vi "RUSHArmControl.vi"(1 "In Cluster":T3) -> (0 "Out Cluster":T2)   [LabVIEW 2012]
uses:
  <vilib>/Rock Robotics/WPI/Relay/WPI_RelayValue.ctl
panel:
  in  "Max Speed":dbl=0.5
  in  "Setpoint P Gain":dbl=2.0
  in  "Manual P Gain":dbl=2.0
  in  "Vision P Gain":dbl=0.75
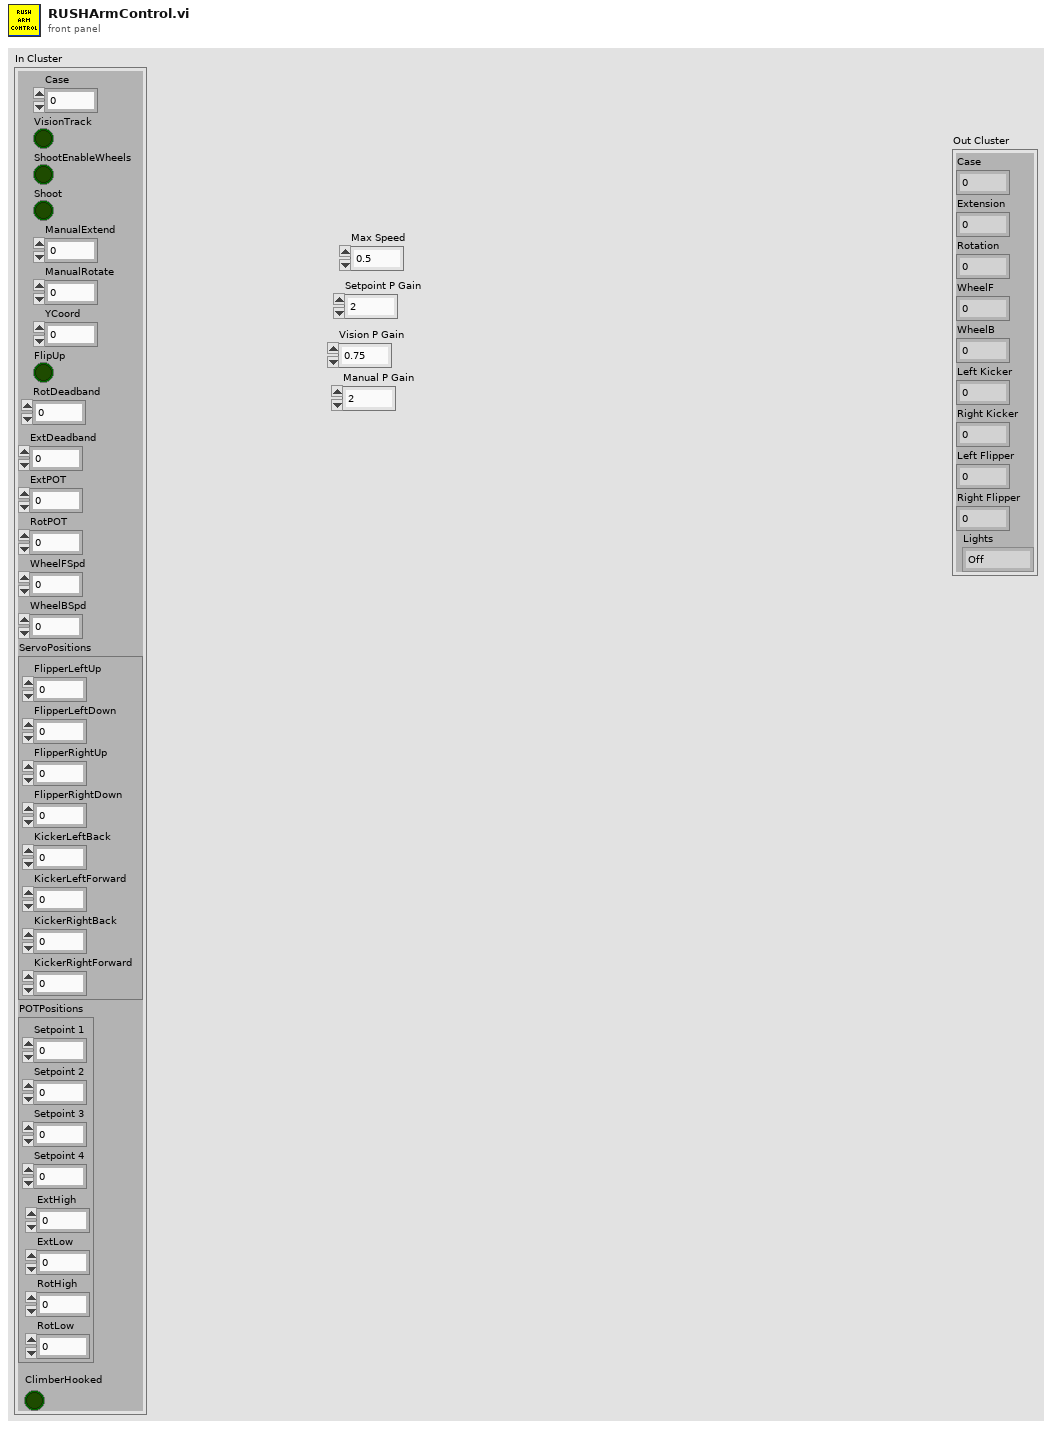
[diagram p1: front panel]
types:
  T1 = typedef "WPI_RelayValue.ctl" = enum16{"Off", "On", "Forward", "Reverse"}
  T2 = cluster{"Case":dbl, "Extension":dbl, "Rotation":dbl, "WheelF":dbl, "WheelB":dbl, "Left Kicker":dbl, "Right Kicker":dbl, "Left Flipper":dbl, "Right Flipper":dbl, "Lights":T1}
  T3 = cluster{"Case":dbl, "VisionTrack":bool, "ShootEnableWheels":bool, "Shoot":bool, "ManualExtend":dbl, "ManualRotate":dbl, "YCoord":dbl, "FlipUp":bool, "RotDeadband":dbl, "ExtDeadband":dbl, "ExtPOT":dbl, "RotPOT":dbl, "WheelFSpd":dbl, "WheelBSpd":dbl, "ServoPositions":cluster{"FlipperLeftUp":dbl, "FlipperLeftDown":dbl, "FlipperRightUp":dbl, "FlipperRightDown":dbl, "KickerLeftBack":dbl, "KickerLeftForward":dbl, "KickerRightBack":dbl, "KickerRightForward":dbl}, "POTPositions":cluster{"Setpoint 1":dbl, "Setpoint 2":dbl, "Setpoint 3":dbl, "Setpoint 4":dbl, "RotLow":dbl, "RotHigh":dbl, "ExtLow":dbl, "ExtHigh":dbl}, "ClimberHooked":bool}
  T4 = cluster{"FlipperLeftUp":dbl, "FlipperLeftDown":dbl, "FlipperRightUp":dbl, "FlipperRightDown":dbl, "KickerLeftBack":dbl, "KickerLeftForward":dbl, "KickerRightBack":dbl, "KickerRightForward":dbl}
  T5 = cluster{"Setpoint 1":dbl, "Setpoint 2":dbl, "Setpoint 3":dbl, "Setpoint 4":dbl, "RotLow":dbl, "RotHigh":dbl, "ExtLow":dbl, "ExtHigh":dbl}
  T6 = cluster{"t":dbl, "y":dbl, "y":dbl, "Output":dbl, "Output":dbl, "KickerLeftBack":dbl, "KickerRightBack":dbl, "FlipperLeftDown":dbl, "FlipperRightDown":dbl, "RelayValue":T1}
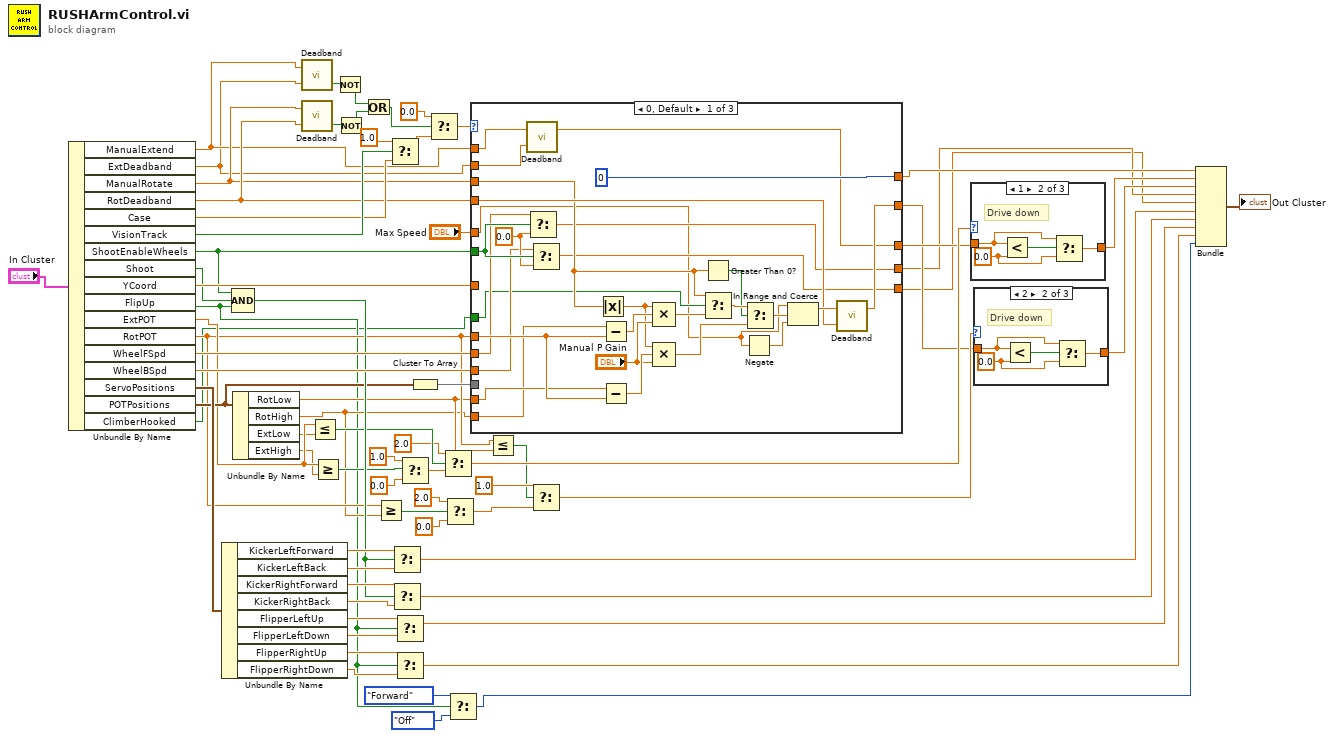
[diagram p0: block diagram]
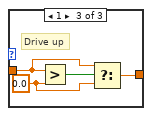
[diagram p3: hidden frame]
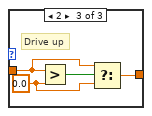
[diagram p5: hidden frame]
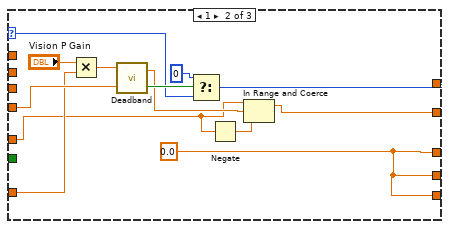
[diagram p6: hidden frame]
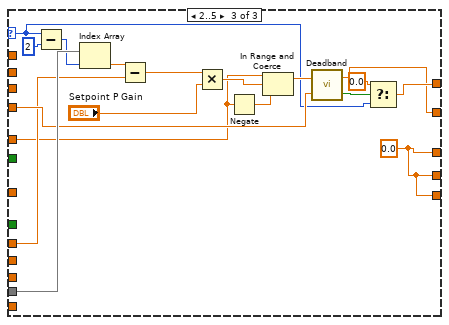
[diagram p7: hidden frame]
diagram:
  n1 = Unbundle By Name("In Cluster") -> ("ManualExtend"=w56:dbl, "ExtDeadband"=w55:dbl, "ManualRotate"=w57:dbl, "RotDeadband"=w59:dbl, "Case"=w60:dbl, "VisionTrack"=w61:bool, "ShootEnableWheels"=w50:bool, "Shoot"=w51:bool, "YCoord"=w58:dbl, "FlipUp"=w6:bool, "ExtPOT"=w33:dbl, "RotPOT"=w21:dbl, "WheelFSpd"=w54:dbl, "WheelBSpd"=w53:dbl, "ServoPositions"=w52:T4, "POTPositions"=w40:T5, "ClimberHooked"=w4:bool)
  n2 = Unbundle By Name(w52) -> ("KickerLeftForward"=w49:dbl, "KickerLeftBack"=w48:dbl, "KickerRightForward"=w47:dbl, "KickerRightBack"=w46:dbl, "FlipperLeftUp"=w44:dbl, "FlipperLeftDown"=w42:dbl, "FlipperRightUp"=w43:dbl, "FlipperRightDown"=w41:dbl)
  n3 = Compound Arithmetic op=AND(w50, w51, w6) -> (w45:bool)
  n4 = Unbundle By Name(w40) -> ("RotLow"=w20:dbl, "RotHigh"=w19:dbl, "ExtLow"=w32:dbl, "ExtHigh"=w31:dbl)
  n5 = call "Deadband.vi"("Deadband"=w55, "Input"=w56) -> ("In Deadband"=w66:bool)  [unwired: 1 out]
  n6 = call "Deadband.vi"("Deadband"=w59, "Input"=w57) -> ("In Deadband"=w65:bool)  [unwired: 1 out]
  n7 = Less Or Equal?(x=w33, y=w32) -> (x <= y?=w34:bool)
  n8 = Greater Or Equal?(x=w33, y=w31) -> (x >= y?=w38:bool)
  n9 = Not(x=w66) -> (.not. x?=w63:bool)
  n10 = Not(x=w65) -> (.not. x?=w64:bool)
  n11 = Or(x=w63, y=w64) -> (x .or. y?=w62:bool)
  n12 = Greater Or Equal?(x=w21, y=w19) -> (x >= y?=w22:bool)
  n13 = Select(t=1.0, s=w61, f=w60) -> (s? t:f=w68:dbl)
  n14 = Select(t=w49, s=w45, f=w48) -> (s? t:f=w11:dbl)
  n15 = Select(t=w47, s=w45, f=w46) -> (s? t:f=w10:dbl)
  n16 = Select(t=w44, s=w6, f=w42) -> (s? t:f=w9:dbl)
  n17 = Select(t=w43, s=w6, f=w41) -> (s? t:f=w8:dbl)
  n18 = Select(t=1.0, s=w38, f=0.0) -> (s? t:f=w35:dbl)
  n19 = Cluster To Array(cluster=w40) -> (array=w39:dbl[])
  n20 = Select(t=0.0, s=w62, f=w68) -> (s? t:f=w71:dbl)
  n21 = Select(t=2.0, s=w34, f=w35) -> (s? t:f=w29:dbl)
  n22 = Select(t=2.0, s=w22, f=0.0) -> (s? t:f=w25:dbl)
  n23 = Select(t=WPI_RelayValue."Forward" ("RelayValue"), s=w6, f=WPI_RelayValue."Off" ("RelayValue")) -> (s? t:f=w2:T1)
  n24 = case shown="0, Default" w71 {
    selector: w71 -> [_ w108 w118]
    tunnel: w59 -> [w86 w111 w122]
    tunnel: w58 -> [_ w110 _]
    tunnel: [0 ("t") w106 w117] -> w16
    tunnel: [w84 w101 w116] -> w17
    tunnel: w21 -> [w89 _ w121]
    tunnel: w20 -> [w88 _ _]
    tunnel: w19 -> [w87 _ _]
    tunnel: w57 -> [w85 _ _]
    tunnel: w56 -> [w82 _ _]
    tunnel: w55 -> [w81 _ _]
    tunnel: [w80 w105 w115] -> w28
    tunnel: w50 -> [w79 _ _]
    tunnel: w54 -> [w77 _ _]
    tunnel: w53 -> [w76 _ _]
    tunnel: [w75 w105 w115] -> w13
    tunnel: [w74 w105 w115] -> w12
    tunnel: w39 -> [_ _ w130]
    tunnel: w4 -> [w73 _ _]
    tunnel: "Max Speed" -> [w72 w102 w114]
    frame 0, Default {
      w78 = 0.0 ("f")
      n25 = call "Deadband.vi"("Deadband"=w81, "Input"=w82) -> ("Output"=w80:dbl)  [unwired: 1 out]
      n26 = Select(t=w77, s=w79, f=w78) -> (s? t:f=w75:dbl)
      n27 = Select(t=w76, s=w79, f=w78) -> (s? t:f=w74:dbl)
      n28 = Absolute Value(x=w85) -> (abs(x)=w94:dbl)
      n29 = Subtract(x=w87, y=w89) -> (x-y=w100:dbl)
      n30 = Subtract(x=w88, y=w89) -> (x-y=w99:dbl)
      n31 = Compound Arithmetic op=MULTIPLY(w94, w100, "Manual P Gain") -> (w97:dbl)
      n32 = Compound Arithmetic op=MULTIPLY(w94, w99, "Manual P Gain") -> (w95:dbl)
      n33 = Greater Than 0?(x=w85) -> (x > 0?=w93:bool)
      n34 = Select(t=w85, s=w73, f=w97) -> (s? t:f=w96:dbl)
      n35 = Negate(x=w72) -> (-x=w91:dbl)
      n36 = Select(t=w96, s=w93, f=w95) -> (s? t:f=w92:dbl)
      n37 = In Range and Coerce(upper limit=w72, x=w92, lower limit=w91) -> (coerced(x)=w90:dbl)  [unwired: 1 out]
      n38 = call "Deadband.vi"("Deadband"=w86, "Input"=w90) -> ("Output"=w84:dbl)  [unwired: 1 out]
    }
    frame 1 {
      w105 = 0.0 ("Output")
      n39 = Multiply(x="Vision P Gain", y=w110) -> (x*y=w112:dbl)
      n40 = call "Deadband.vi"("Deadband"=w111, "Input"=w112) -> ("In Deadband"=w109:bool, "Output"=w103:dbl)
      n41 = Select(t=0, s=w109, f=w108) -> (s? t:f=w106:i32)
      n42 = Negate(x=w102) -> (-x=w104:dbl)
      n43 = In Range and Coerce(upper limit=w102, x=w103, lower limit=w104) -> (coerced(x)=w101:dbl)  [unwired: 1 out]
    }
    frame 2..5 {
      w115 = 0.0 ("Output")
      n44 = Subtract(x=w118, y=2) -> (x-y=w129:i32)
      n45 = Index Array(array=w130, index=w129) -> (element=w128:dbl)
      n46 = Subtract(x=w128, y=w121) -> (x-y=w127:dbl)
      n47 = Multiply(x=w127, y="Setpoint P Gain") -> (x*y=w124:dbl)
      n48 = Negate(x=w114) -> (-x=w125:dbl)
      n49 = In Range and Coerce(upper limit=w114, x=w124, lower limit=w125) -> (coerced(x)=w123:dbl)  [unwired: 1 out]
      n50 = call "Deadband.vi"("Deadband"=w122, "Input"=w123) -> ("In Deadband"=w120:bool, "Output"=w116:dbl)
      n51 = Select(t=0.0, s=w120, f=w118) -> (s? t:f=w117:dbl)
    }
  }
  n52 = Less Or Equal?(x=w21, y=w20) -> (x <= y?=w26:bool)
  n53 = Select(t=1.0, s=w26, f=w25) -> (s? t:f=w18:dbl)
  n54 = case shown="1" w29 {
    tunnel: w28 -> [w132 w134 w138]
    tunnel: [w132 w133 w137] -> w15
    frame 0, Default {
      # "All good"
    }
    frame 1 {
      w135 = 0.0 ("y")
      # "Drive down"
      n55 = Less?(x=w134, y=w135) -> (x < y?=w136:bool)
      n56 = Select(t=w134, s=w136, f=w135) -> (s? t:f=w133:dbl)
    }
    frame 2 {
      w139 = 0.0 ("y")
      # "Drive up"
      n57 = Greater?(x=w138, y=w139) -> (0:w140:bool)
      n58 = Select(t=w138, s=w140, f=w139) -> (s? t:f=w137:dbl)
    }
  }
  n59 = case shown="2" w18 {
    tunnel: w17 -> [w141 w143 w147]
    tunnel: [w141 w142 w146] -> w14
    frame 0, Default {
      # "All good"
    }
    frame 2 {
      w144 = 0.0 ("y")
      # "Drive down"
      n60 = Less?(x=w143, y=w144) -> (x < y?=w145:bool)
      n61 = Select(t=w143, s=w145, f=w144) -> (s? t:f=w142:dbl)
    }
    frame 1 {
      w148 = 0.0 ("y")
      # "Drive up"
      n62 = Greater?(x=w147, y=w148) -> (0:w149:bool)
      n63 = Select(t=w147, s=w149, f=w148) -> (s? t:f=w146:dbl)
    }
  }
  n64 = Bundle("t"=w16, "y"=w15, "y"=w14, "Output"=w13, "Output"=w12, "KickerLeftBack"=w11, "KickerRightBack"=w10, "FlipperLeftDown"=w9, "FlipperRightDown"=w8, "RelayValue"=w2) -> (→"Out Cluster":T6)  [unwired: 1 in]
